vi "AcquisitionLoop_Simplified.vi"(8 "error in":errorcluster, 10 "Image Queue":refnum<queue>, 11 "Loop State Queue":refnum<queue>) -> (0 "error out":errorcluster)   [LabVIEW 2017, in "ImageAcquisitionLibrary.lvlib"]
uses:
  ImageAcquisitionLibrary.lvlib
  AcquisitionLoopState.ctl
  AcquireData.ctl
  AcquisitionObject.ctl
  <vilib>/vision/Image Controls.llb/IMAQ Image.ctl
  Settings/Settings.ctl
  <vilib>/userdefined/High Color/IMAQdx.ctl
  Tracking/TrackingSettings.ctl
  Settings/Calibration.ctl
  <vilib>/Utility/error.llb/DialogType.ctl
  SettingsGlobal.vi
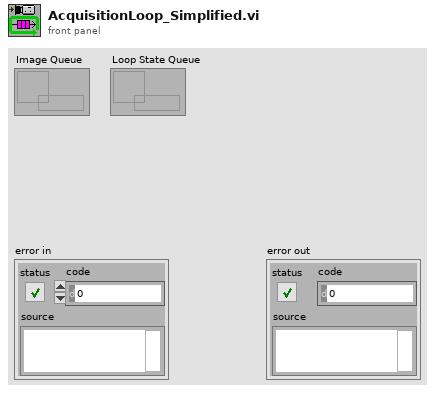
[diagram p1: front panel]
types:
  T1 = typedef "ImageAcquisitionLibrary.lvlib/Settings.ctl" = cluster{"Harware Configuration":cluster{"Camera":T2, "Frames Per Second":u32, "Simulate Recording":bool, "Simulated Recording Sample":path, "Timestamp Method":enum16{"System Timestamp", "Camera Timestamp", "IMAQdx Timestamp"}}, "Base Recording Path":path, "Type Of Recording":string, "Recording Codec":string, "TrackingSettings":T3, "Calibration":T5, "Broadcast Length":i32}
  T2 = typedef "IMAQdx.ctl" = refnum<k21>
  T3 = typedef "ImageAcquisitionLibrary.lvlib/TrackingSettings.ctl" = cluster{"Max Radius":i32, "Threshold":sgl, "ROI":T4}
  T4 = typedef "IMAQ Rectangle" = cluster{"Left":i32, "Top":i32, "Right":i32, "Bottom":i32, "Rotation":dbl}
  T5 = typedef "ImageAcquisitionLibrary.lvlib/Calibration.ctl" = cluster{"Pixel Width (X)":dbl, "Pixel Height (Y)":dbl}
  T6 = typedef "ImageAcquisitionLibrary.lvlib/AcquireData.ctl" = cluster{"Frame Data":cluster{"Image":u32[][], "Timestamp":timestamp, "Image Type":T7, "Dropped Frames":u32}, "Tracking Data":cluster{"Positions":dbl[][], "Timestamp":timestamp}, "Tracked?":bool}
  T7 = typedef "Image Type" = u32
  T8 = typedef "ImageAcquisitionLibrary.lvlib/AcquisitionObject.ctl" = cluster{"Camera Session":T9, "Last Frame":u32, "Dropped Frames":u32, "Image Type":T7}
  T9 = typedef "IMAQ Image.ctl" = refnum<image>
  T10 = typedef "ImageAcquisitionLibrary.lvlib/AcquisitionLoopState.ctl" = enum16{"Start Acquisition", "Acquire", "Stop Acquisition", "Update Settings", "Exit"}
  T11 = typedef "DialogType.ctl" = u16
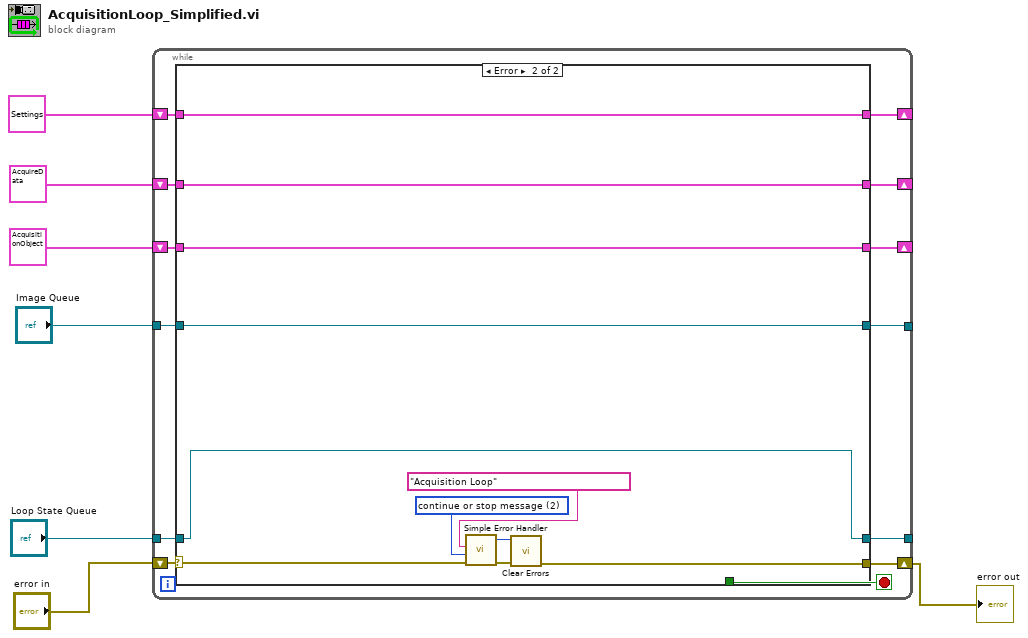
[diagram p0: block diagram]
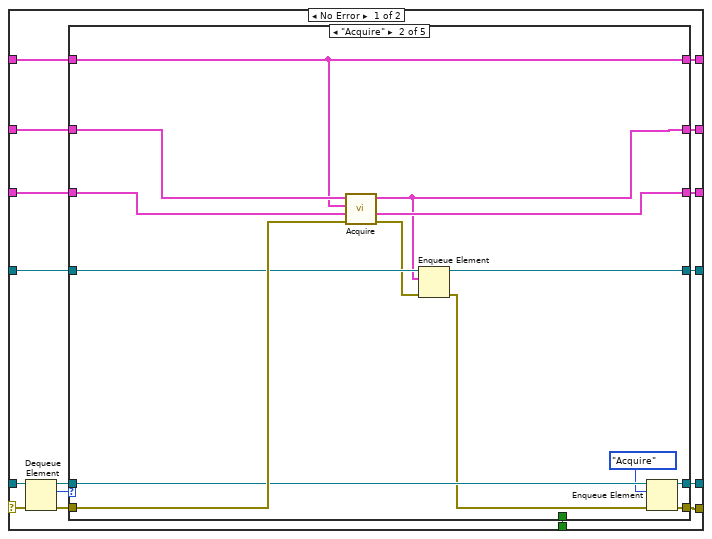
[diagram p2: hidden frame]
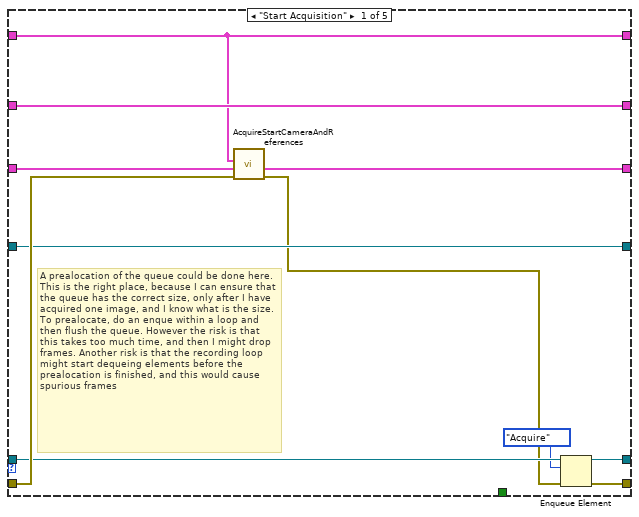
[diagram p3: hidden frame]
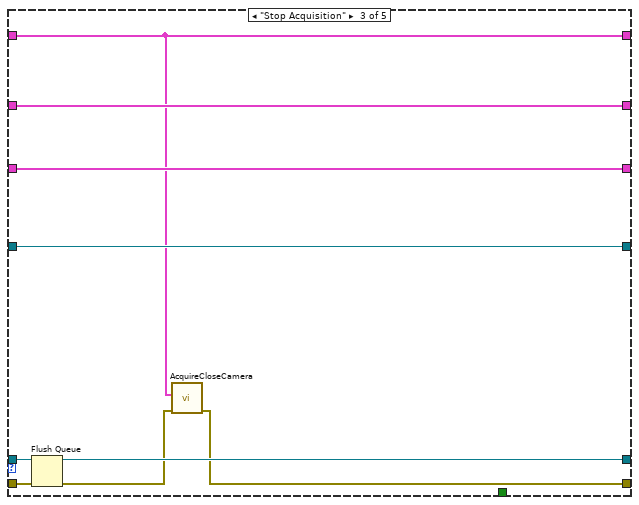
[diagram p4: hidden frame]
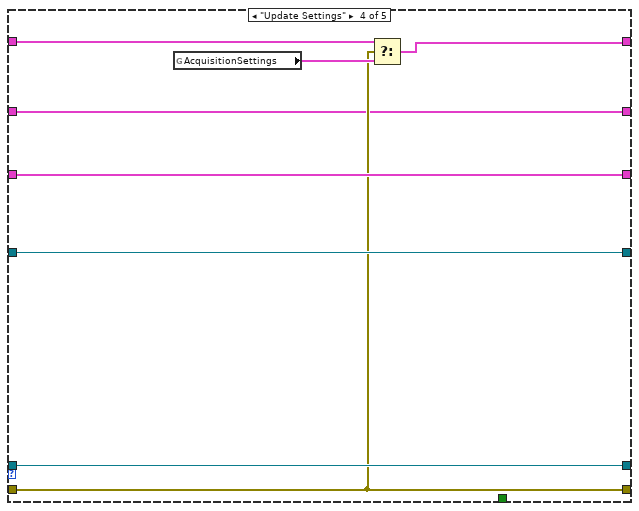
[diagram p5: hidden frame]
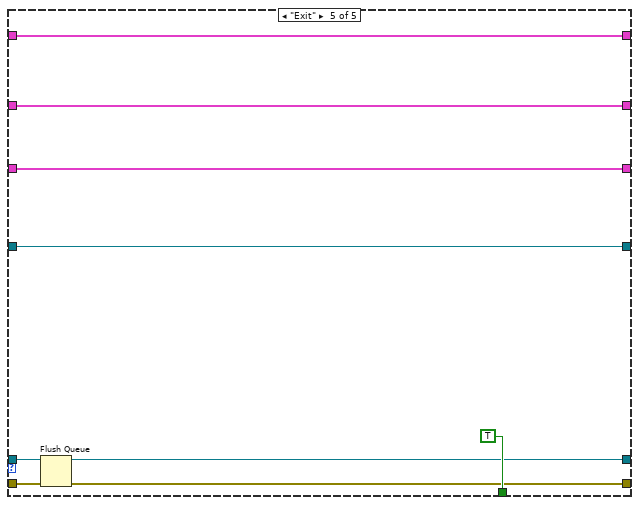
[diagram p6: hidden frame]
diagram:
  n1 = while {
    tunnel: [w17] -> _
    tunnel: "Image Queue" -> [w16]
    shift-right: [w14] -> _
    shift-left: T6 {"Frame Data"={"Image"=[], "Timestamp"=timestamp(0 s since 1904-01-01), "Image Type"=0, "Dropped Frames"=0}, "Tracking Data"={"Positions"=[], "Timestamp"=timestamp(0 s since 1904-01-01)}, "Tracked?"=FALSE} ("Acquired Data") -> [w15]
    shift-right: [w12] -> _
    shift-left: T8 {"Camera Session"=refnum, "Last Frame"=0, "Dropped Frames"=0, "Image Type"=0} -> [w13]
    tunnel: "Loop State Queue" -> [w11]
    tunnel: [w10] -> _
    shift-right: [w9] -> _
    shift-left: T1 {"Harware Configuration"={"Camera"="cam1", "Frames Per Second"=15, "Simulate Recording"=FALSE, "Simulated Recording Sample"=path "", "Timestamp Method"=enum."Camera Timestamp"}, "Base Recording Path"=path "", "Type Of Recording"="", "Recording Codec"="", "TrackingSettings"={"Max Radius"=0, "Threshold"=160.0, "ROI"={"Left"=0, "Top"=0, "Right"=0, "Bottom"=0, "Rotation"=0.0}}, "Calibration"={"Pixel Width (X)"=10.0, "Pixel Height (Y)"=100.0}, "Broadcast Length"=0} ("Settings") -> [w8]
    shift-right: [w18] -> w5
    shift-left: "error in" -> [w20]
    stop <- w19 stop-if-true
    n2 = case shown="Error" w20 {
      selector: w20 -> [w27 w96]
      tunnel: [w36 _] -> w19
      tunnel: [w35 w95] -> w18
      tunnel: [w29 w92] -> w17
      tunnel: w16 -> [w34 w92]
      tunnel: w15 -> [w33 w91]
      tunnel: [w32 w91] -> w14
      tunnel: w13 -> [w31 w90]
      tunnel: [w30 w90] -> w12
      tunnel: w11 -> [w28 w89]
      tunnel: [w23 w89] -> w10
      tunnel: [w22 w88] -> w9
      tunnel: w8 -> [w21 w88]
      frame No Error {
        n3 = Dequeue Element(queue=w28, error in (no error)=w27) -> (queue out=w24:refnum<queue>, element=w25:T10, error out=w26:errorcluster)  [unwired: 1 in, 1 out]
        n4 = case shown="\"Acquire\"" w25 {
          tunnel: [_ _ _ _ TRUE] -> w36
          tunnel: w26 -> [w45 w60 w70 w74 w85]
          tunnel: [w44 w52 w66 w74 w84] -> w35
          tunnel: w34 -> [w40 w57 w65 w77 w86]
          tunnel: w33 -> [w38 w61 w63 w73 w81]
          tunnel: [w38 w49 w63 w73 w81] -> w32
          tunnel: w31 -> [w46 w59 w64 w78 w80]
          tunnel: [w47 w58 w64 w78 w80] -> w30
          tunnel: [w40 w56 w65 w77 w86] -> w29
          tunnel: w24 -> [w42 w54 w69 w76 w83]
          tunnel: [w43 w53 w68 w76 w82] -> w23
          tunnel: [w37 w50 w62 w71 w79] -> w22
          tunnel: w21 -> [w37 w50 w62 w72 w79]
          frame "Start Acquisition" {
            # "A prealocation of the queue could be done here. This is the right place, because I can ensure that the queue has the correct size, only after I have acquired one image, and I know what is the size. \nTo prealocate, do an enque within a loop and then flush the queue. However the risk is that this takes too much time, and then I might drop frames. Another risk is that the recording loop might start dequeing elements before the prealocation is finished, and this would cause spurious frames"
            n5 = call "AcquireStartCameraAndReferences.vi"("error in (no error)"=w45, 9:w46, "Settings"=w37) -> ("error out"=w39:errorcluster, 1:w47:T8)  [unwired: 7 in]
            n6 = Enqueue Element(queue=w42, element=AcquisitionLoopState."Acquire", error in (no error)=w39) -> (queue out=w43:refnum<queue>, error out=w44:errorcluster)  [unwired: 1 in, 1 out]
          }
          frame "Acquire" {
            n7 = call "Acquire.vi"("error in (no error)"=w60, 9:w59, "Settings"=w50, "Acquired Data"=w61) -> ("error out"=w55:errorcluster, "Acquisition Object"=w58:T8, "Acquired Data out"=w49:T6)  [unwired: 5 in]
            n8 = Enqueue Element(queue=w57, element=w49, error in (no error)=w55) -> (queue out=w56:refnum<queue>, error out=w48:errorcluster)  [unwired: 1 in, 1 out]
            n9 = Enqueue Element(queue=w54, element=AcquisitionLoopState."Acquire", error in (no error)=w48) -> (queue out=w53:refnum<queue>, error out=w52:errorcluster)  [unwired: 1 in, 1 out]
          }
          frame "Stop Acquisition" {
            n10 = Flush Queue(queue=w69, error in (no error)=w70) -> (queue out=w68:refnum<queue>, error out=w67:errorcluster)  [unwired: 1 out]
            n11 = call "AcquireCloseCamera.vi"("error in (no error)"=w67, "Settings"=w62) -> ("error out"=w66:errorcluster)  [unwired: 9 in]
          }
          frame "Update Settings" {
            n12 = global read "SettingsGlobal.vi" "AcquisitionSettings"() -> (w75:T1)
            n13 = Select(t=w72, s=w74, f=w75) -> (s? t:f=w71:T1)
          }
          frame "Exit" {
            n14 = Flush Queue(queue=w83, error in (no error)=w85) -> (queue out=w82:refnum<queue>, error out=w84:errorcluster)  [unwired: 1 out]
          }
        }
      }
      frame Error {
        w93 = T11 2 items=["no dialog", "OK message", "continue or stop message", "OK message + warnings", "continue/stop + warnings"] ("type of dialog (OK msg:1)")
        n15 = call <vilib>:"Simple Error Handler.vi"("error source (\" \")"="Acquisition Loop" ("error source (\" \")"), "type of dialog (OK msg:1)"=w93, "error in (no error)"=w96) -> ("code out"=w97:i32, "error out"=w98:errorcluster)  [unwired: 2 in, 3 out]
        n16 = call <vilib>:"Clear Errors.vi"("error in (no error)"=w98, "specific error code to clear (0: all)"=w97) -> ("error out"=w95:errorcluster)  [unwired: 4 in, 1 out]
      }
    }
  }
  "error out" <- w5
